vi "Get DLL Path.vi"() -> (2 "Path":path)   [LabVIEW 2015, in "JSON Document.lvclass"]
uses:
  API/JSON Document Class/JSON Document.lvclass
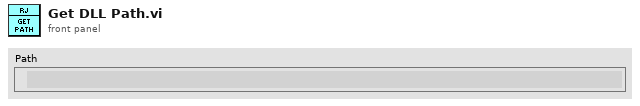
[diagram p1: front panel]
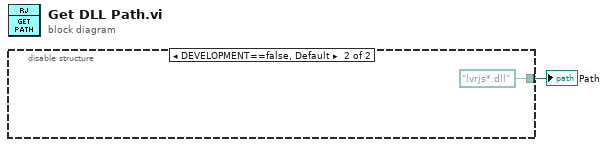
[diagram p0: block diagram]
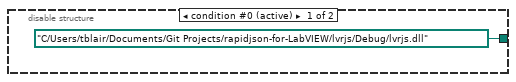
[diagram p2: hidden frame]
diagram:
  n1 = disable-structure shown="DEVELOPMENT==false, Default" {
    disable-tunnel: [path "C:/Users/tblair/Documents/Git Projects/rapidjson-for-LabVIEW/lvrjs/Debug/lvrjs.dll" path "lvrjs*.dll" ("Path")] -> w1
    frame condition #0 (active) {
    }
    frame condition #1 {
    }
  }
  "Path" <- w1
